vi "ALTS-2015 Update Start Stop DO.vi"(7 "DO Options":T1, 8 "error in":errorcluster, 11 "Station Cluster":T2) -> (0 "error out":errorcluster)   [LabVIEW 2013]
uses:
  Controls/ALTS-2015 Station Cluster.ctl
  Controls/ALTS-2015 DO Start Stop Options.ctl
  SLL DAQ Engine/Software/Source Code/Sub VIs/DAQ Engine/Controls/SLL DE DO Global Options.ctl
  SLL DAQ Engine/Software/Source Code/Sub VIs/DAQ Engine/Controls/SLL DE List of Digital Outputs.ctl
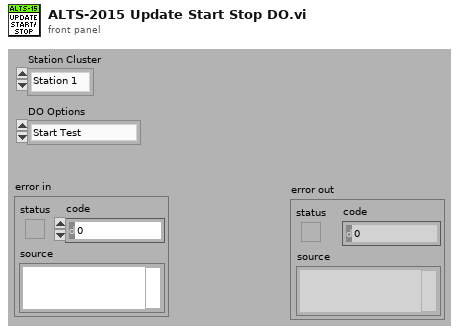
[diagram p1: front panel]
types:
  T1 = typedef "ALTS-2015 DO Start Stop Options.ctl" = enum16{"Start Test", "Stop Test"}
  T2 = typedef "ALTS-2015 Station Cluster.ctl" = enum16{"Station 1", "Station 2", "Station 3", "Station 4"}
  T3 = typedef "SLL DE DO Global Options.ctl" = enum16{"Init", "Write Line", "Write Array", "Write Full Status", "Read Line", "Read Array", "Read Full Status", "Restart DO", "Send to Safe Mode", "Stop DO"}
  T4 = typedef "SLL DE List of Digital Outputs.ctl" = enum16{"STATION1_START TEST", "STATION1_STOP TEST", "STATION1_LIGHT1", "STATION1_LIGHT2", "STATION1_LIGHT3", "STATION1_SELECT_TEST", "STATION2_START TEST", "STATION2_STOP TEST", "STATION2_LIGHT1", "STATION2_LIGHT2", "STATION2_LIGHT3", "STATION2_SELECT_TEST", "STATION3_START TEST", "STATION3_STOP TEST", "STATION3_LIGHT1", "STATION3_LIGHT2", "STATION3_LIGHT3", "STATION3_SELECT_TEST", "STATION4_START TEST", "STATION4_STOP TEST", "STATION4_LIGHT1", "STATION4_LIGHT2", "STATION4_LIGHT3", "STATION4_SELECT_TEST"}
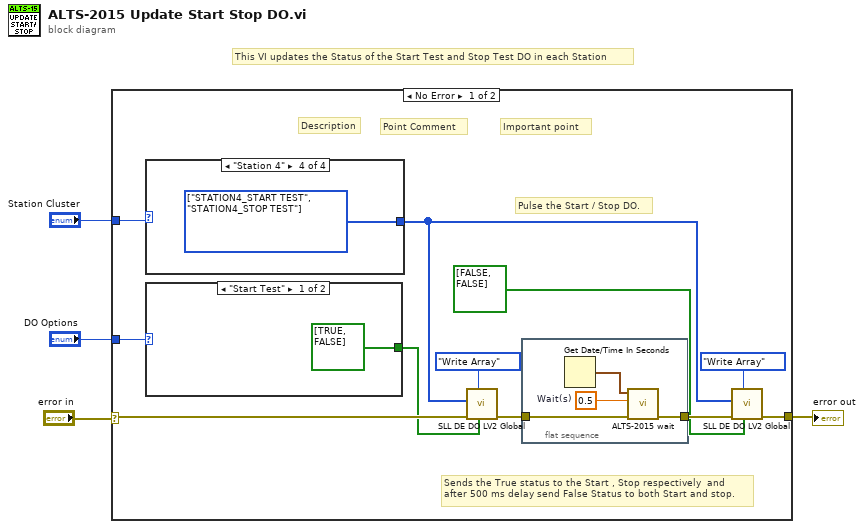
[diagram p0: block diagram]
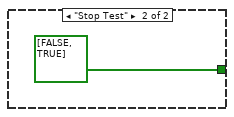
[diagram p2: hidden frame]
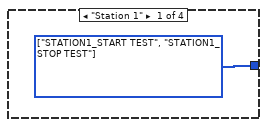
[diagram p3: hidden frame]
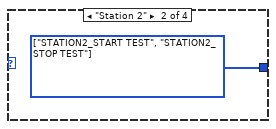
[diagram p4: hidden frame]
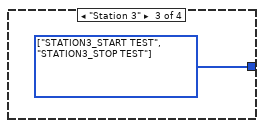
[diagram p5: hidden frame]
diagram:
  # "This VI updates the Status of the Start Test and Stop Test DO in each Station"
  n1 = case shown="No Error" "error in" {
    selector: "error in" -> [w13 w26]
    tunnel: "DO Options" -> [w12 _]
    tunnel: [w8 w26] -> w4
    tunnel: "Station Cluster" -> [w15 _]
    frame No Error {
      # "Sends the True status to the Start , Stop respectively  and \nafter 500 ms delay send False Status to both Start and stop."
      # "Point Comment"
      # "Important point"
      # "Description"
      # "Pulse the Start / Stop DO."
      n2 = case shown="\"Station 4\"" w15 {
        tunnel: [w22 w23 w24 w25] -> w9
        frame "Station 1" {
          w22 = T4[] [enum."STATION1_START TEST", enum."STATION1_STOP TEST"] items=["STATION1_START TEST", "STATION1_STOP TEST", "STATION1_LIGHT1", "STATION1_LIGHT2", "STATION1_LIGHT3", "STATION1_SELECT_TEST", "STATION2_START TEST", "STATION2_STOP TEST", "STATION2_LIGHT1", "STATION2_LIGHT2", "STATION2_LIGHT3", "STATION2_SELECT_TEST", "STATION3_START TEST", "STATION3_STOP TEST", "STATION3_LIGHT1", "STATION3_LIGHT2", "STATION3_LIGHT3", "STATION3_SELECT_TEST", "STATION4_START TEST", "STATION4_STOP TEST", "STATION4_LIGHT1", "STATION4_LIGHT2", "STATION4_LIGHT3", "STATION4_SELECT_TEST"] ("DO Channel Name Array")
        }
        frame "Station 2" {
          w23 = T4[] [enum."STATION2_START TEST", enum."STATION2_STOP TEST"] items=["STATION1_START TEST", "STATION1_STOP TEST", "STATION1_LIGHT1", "STATION1_LIGHT2", "STATION1_LIGHT3", "STATION1_SELECT_TEST", "STATION2_START TEST", "STATION2_STOP TEST", "STATION2_LIGHT1", "STATION2_LIGHT2", "STATION2_LIGHT3", "STATION2_SELECT_TEST", "STATION3_START TEST", "STATION3_STOP TEST", "STATION3_LIGHT1", "STATION3_LIGHT2", "STATION3_LIGHT3", "STATION3_SELECT_TEST", "STATION4_START TEST", "STATION4_STOP TEST", "STATION4_LIGHT1", "STATION4_LIGHT2", "STATION4_LIGHT3", "STATION4_SELECT_TEST"] ("DO Channel Name Array")
        }
        frame "Station 3" {
          w24 = T4[] [enum."STATION3_START TEST", enum."STATION3_STOP TEST"] items=["STATION1_START TEST", "STATION1_STOP TEST", "STATION1_LIGHT1", "STATION1_LIGHT2", "STATION1_LIGHT3", "STATION1_SELECT_TEST", "STATION2_START TEST", "STATION2_STOP TEST", "STATION2_LIGHT1", "STATION2_LIGHT2", "STATION2_LIGHT3", "STATION2_SELECT_TEST", "STATION3_START TEST", "STATION3_STOP TEST", "STATION3_LIGHT1", "STATION3_LIGHT2", "STATION3_LIGHT3", "STATION3_SELECT_TEST", "STATION4_START TEST", "STATION4_STOP TEST", "STATION4_LIGHT1", "STATION4_LIGHT2", "STATION4_LIGHT3", "STATION4_SELECT_TEST"] ("DO Channel Name Array")
        }
        frame "Station 4" {
          w25 = T4[] [enum."STATION4_START TEST", enum."STATION4_STOP TEST"] items=["STATION1_START TEST", "STATION1_STOP TEST", "STATION1_LIGHT1", "STATION1_LIGHT2", "STATION1_LIGHT3", "STATION1_SELECT_TEST", "STATION2_START TEST", "STATION2_STOP TEST", "STATION2_LIGHT1", "STATION2_LIGHT2", "STATION2_LIGHT3", "STATION2_SELECT_TEST", "STATION3_START TEST", "STATION3_STOP TEST", "STATION3_LIGHT1", "STATION3_LIGHT2", "STATION3_LIGHT3", "STATION3_SELECT_TEST", "STATION4_START TEST", "STATION4_STOP TEST", "STATION4_LIGHT1", "STATION4_LIGHT2", "STATION4_LIGHT3", "STATION4_SELECT_TEST"] ("DO Channel Name Array")
        }
      }
      n3 = case shown="\"Start Test\"" w12 {
        tunnel: [bool[] [TRUE, FALSE] ("DO State Array") bool[] [FALSE, TRUE] ("DO State Array")] -> w11
        frame "Start Test" {
        }
        frame "Stop Test" {
        }
      }
      n4 = call "SLL DE DO LV2 Global.vi"("DO State Array"=w11, "DO Option"=SLL_DE_DO_Global_Options."Write Array", "Error In"=w13, "DO Channel Name Array"=w9) -> ("error out"=w7:errorcluster)  [unwired: 4 in, 3 out]
      n5 = flat-sequence {
        tunnel: w7 -> [w17]
        tunnel: [w16] -> w6
        frame #0 {
          w18 = 0.5  # Wait(s)
          n6 = Get Date/Time In Seconds() -> (seconds since 1Jan1904=w19:timestamp)
          n7 = call "ALTS-2015 wait.vi"("error in"=w17, "Wait (s)"=w18, "Start time"=w19) -> ("error out"=w16:errorcluster)  [unwired: 6 in, 2 out]
        }
      }
      n8 = call "SLL DE DO LV2 Global.vi"("DO State Array"=bool[] [FALSE, FALSE], "DO Option"=SLL_DE_DO_Global_Options."Write Array", "Error In"=w6, "DO Channel Name Array"=w9) -> ("error out"=w8:errorcluster)  [unwired: 4 in, 3 out]
    }
    frame Error {
    }
  }
  "error out" <- w4
